vi "Save To File.vi"(8 "error in (no error)":errorcluster, 10 "Sudoku File":path, 11 "Sudoku String":T1) -> (0 "error out":errorcluster)   [LabVIEW 2015, in "Sudoku Library.lvlib"]
doc: "Created IvanLis by LabVIEW Portal\nProfile: http://labviewportal.org/memberlist.php?mode=viewprofile&u=987\neMail: IvanLisanov@gMail.com\nTelegram: https://t.me/IvanLis"
uses:
  Sudoku Library.lvlib
  TypeDef/Sudoku String.ctl
  <vilib>/Utility/file.llb/Write Delimited Spreadsheet (string).vi
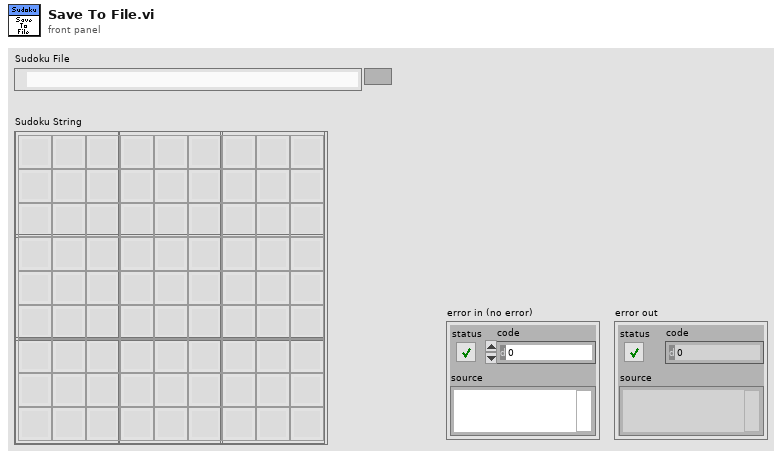
[diagram p1: front panel]
types:
  T1 = typedef "Sudoku Library.lvlib/Sudoku String.ctl" = string[][]
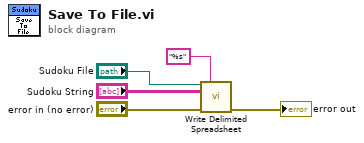
[diagram p0: block diagram]
diagram:
  n1 = call-poly <vilib>:"Write Delimited Spreadsheet.vi"("file path (dialog if empty)"="Sudoku File", "format (%s)"="%s" ("format (%.3f)"), "2D data"="Sudoku String", "error in (no error)"="error in (no error)") -> ("error out"=→"error out":errorcluster)  [unwired: 10 in, 1 out]
